vi "VolumeCoordinate.vi"(9 "NumPoints":u32, 10 "SampleNum":u32, 11 "Scan Settings":T1) -> (1 "PointNum":u32, 2 "RepNum":u32, 3 "Point":cluster{"X":i32, "Y":i32, "Z":i32})   [LabVIEW 2014]
uses:
  <vilib>/rvi/Emulation/niFpgaSctlEmulationGetInTimedLoop.vi
  <vilib>/rvi/Emulation/niFpgaProcessEmulError.vi
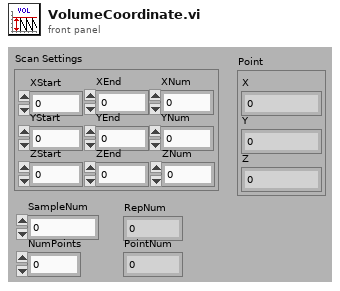
[diagram p1: front panel]
types:
  T1 = cluster{"XStart":i32, "XEnd":i32, "XNum":i32, "YStart":i32, "YEnd":i32, "YNum":i32, "ZStart":i32, "ZEnd":i32, "ZNum":i32}
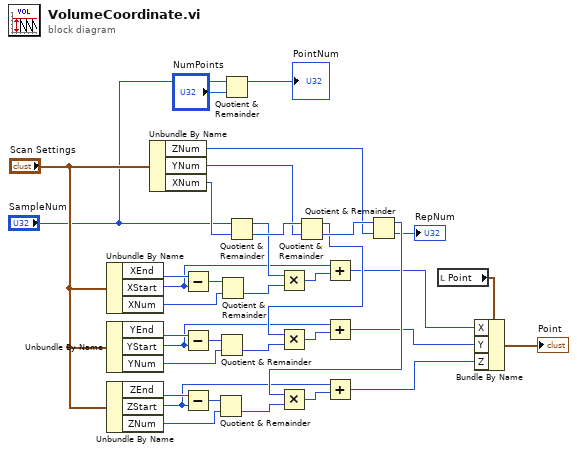
[diagram p0: block diagram]
diagram:
  n1 = Unbundle By Name("Scan Settings") -> ("XEnd"=w29:i32, "XStart"=w10:i32, "XNum"=w12:i32)
  n2 = Unbundle By Name("Scan Settings") -> ("YEnd"=w27:i32, "YStart"=w9:i32, "YNum"=w15:i32)
  n3 = Unbundle By Name("Scan Settings") -> ("ZEnd"=w23:i32, "ZStart"=w8:i32, "ZNum"=w18:i32)
  n4 = Unbundle By Name("Scan Settings") -> ("ZNum"=w4:i32, "YNum"=w5:i32, "XNum"=w6:i32)
  n5 = Subtract(x=w29, y=w10) -> (x-y=w13:i32)
  n6 = Subtract(x=w27, y=w9) -> (x-y=w16:i32)
  n7 = Subtract(x=w23, y=w8) -> (x-y=w19:i32)
  n8 = Quotient & Remainder(x=w19, y=w18) -> (floor(x/y)=w17:i32)  [unwired: 1 out]
  n9 = Quotient & Remainder(x=w16, y=w15) -> (floor(x/y)=w14:i32)  [unwired: 1 out]
  n10 = Quotient & Remainder(x=w13, y=w12) -> (floor(x/y)=w11:i32)  [unwired: 1 out]
  n11 = Quotient & Remainder(x="SampleNum", y="NumPoints") -> (x-y*floor(x/y)=→"PointNum":u32)  [unwired: 1 out]
  n12 = Quotient & Remainder(x="SampleNum", y=w6) -> (x-y*floor(x/y)=w31:u32, floor(x/y)=w36:u32)
  n13 = Multiply(x=w31, y=w11) -> (x*y=w30:u32)
  n14 = Quotient & Remainder(x=w36, y=w5) -> (x-y*floor(x/y)=w26:u32, floor(x/y)=w35:u32)
  n15 = Multiply(x=w26, y=w14) -> (x*y=w28:u32)
  n16 = Add(x=w10, y=w30) -> (x+y=w22:u32)
  n17 = Add(x=w9, y=w28) -> (x+y=w21:u32)
  n18 = Quotient & Remainder(x=w35, y=w4) -> (x-y*floor(x/y)=w24:u32, floor(x/y)=→"RepNum":u32)
  n19 = Multiply(x=w24, y=w17) -> (x*y=w25:u32)
  n20 = Add(x=w8, y=w25) -> (x+y=w20:u32)
  n21 = local read "Point"() -> (w34:cluster{"X":i32, "Y":i32, "Z":i32})
  n22 = Bundle By Name(cluster=w34, "X"=w22, "Y"=w21, "Z"=w20) -> (→"Point":cluster{"X":i32, "Y":i32, "Z":i32})
